vi "null.vi"(1 "Exit Loop ID":i32=-1, 2 "This Loop ID":i32) -> ()   [LabVIEW 2014]
doc: "Null state VI - does nothing for one iteration (it'll set its own exit value to TRUE) and can optionally end a parallel loops's substate."
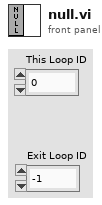
[diagram p1: front panel]
types:
  T1 = typedef "subStates.ctl" = enum16{"null", "wait", "driver control", "auto", "manual override", "hold position", "rotate", "test", "end"}
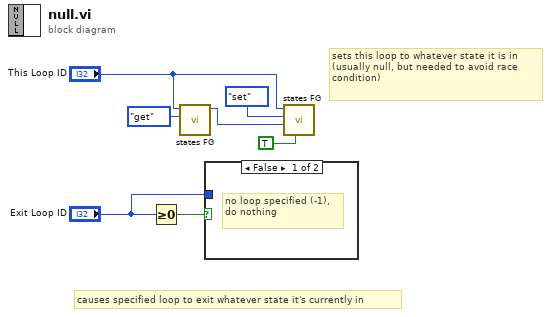
[diagram p0: block diagram]
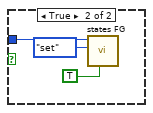
[diagram p2: hidden frame]
diagram:
  # "sets this loop to whatever state it is in\n(usually null, but needed to avoid race \ncondition)"
  # "causes specified loop to exit whatever state it's currently in"
  n1 = Greater Or Equal To 0?(x="Exit Loop ID") -> (x >= 0?=w4:bool)
  n2 = call "states FG.vi"("menu (get)"=enum16{"set", "get"}."get", "Loop ID"="This Loop ID") -> ("subState out"=w3:T1)  [unwired: 6 in, 3 out]
  n3 = case shown="False" w4 {
    tunnel: "Exit Loop ID" -> [_ w8]
    frame False {
      # "no loop specified (-1),\ndo nothing"
    }
    frame True {
      n4 = call "states FG.vi"("exit in"=TRUE, "menu (get)"=enum16{"set", "get"}."set", "Loop ID"=w8) -> ()  [unwired: 5 in, 4 out]
    }
  }
  n5 = call "states FG.vi"("exit in"=TRUE, "subState in"=w3, "menu (get)"=enum16{"set", "get"}."set", "Loop ID"="This Loop ID") -> ()  [unwired: 4 in, 4 out]
